vi "Device_Measurement_Retrieve.vi"(3 "IP Address":string) -> (1 "Measurment Active":bool)   [LabVIEW 2024]
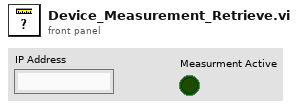
[diagram p1: front panel]
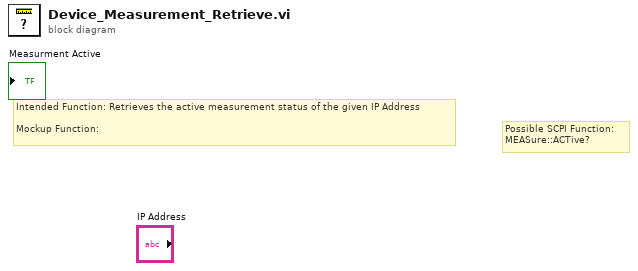
[diagram p0: block diagram]
diagram:
  # "Possible SCPI Function:\nMEASure::ACTive?"
  # "Intended Function: Retrieves the active measurement status of the given IP Address\n\nMockup Function:"
